vi "Output Enable Write Array.vi"(8 "error in":errorcluster, 10 "Output Enable STS":i32[](array[numeric]), 11 "Cycler in":refnum<class "Cycler.lvclass">) -> (0 "error out":errorcluster, 3 "Cycler out":refnum<class "Cycler.lvclass">)   [LabVIEW 2023, in "Cycler.lvclass"]
uses:
  Cycler.lvclass
  Cycler.lvclass/Cycler.ctl
  Low Level Capabilities/Output Enable/Output Enable.lvclass
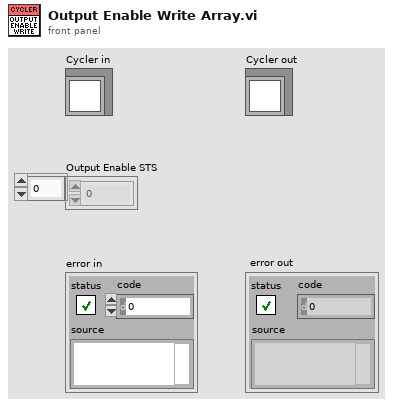
[diagram p1: front panel]
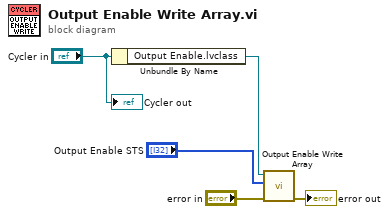
[diagram p0: block diagram]
diagram:
  n1 = Unbundle By Name("Cycler in") -> ("Output Enable.lvclass"=w5:refnum<class "Output Enable.lvclass">)
  n2 = call-dynamic "Output Enable Write Array.vi"("error in"="error in", "Output Enable STS"="Output Enable STS", "Output Enable in"=w5) -> ("error out"=→"error out":errorcluster)  [unwired: 7 in, 1 out]
  "Cycler out" <- "Cycler in"
